vi "IncrementOldHandleMutation.vi"(4 "SerializableData_v2.ctl":path, 6 "Mutate_v1_to_v2.vi":path, 8 "error in (no error)":errorcluster, 10 "Application":refnum<vi>, 11 "LVClassLibrary Ref":refnum<vi>) -> (0 "error out":errorcluster, 2 "Application":refnum<vi>, 3 "LVClassLibrary Ref":refnum<vi>)   [LabVIEW 2019, in "BlueSerializationScripts.lvlib"]
uses:
  BlueSerializationScripts.lvlib
  <userlib>/_OpenG.lib/file/file.llb/File Exists - Scalar__ogtk.vi
  BlueSerialProviderGlobal.vi
  BlueUtilityScripts/BlueUtilityScripts.lvlib
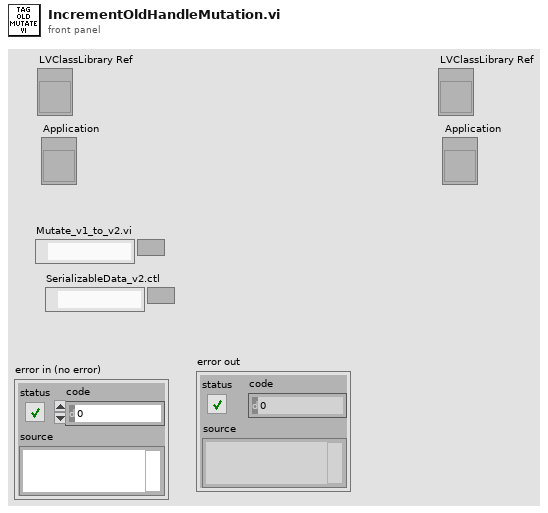
[diagram p1: front panel]
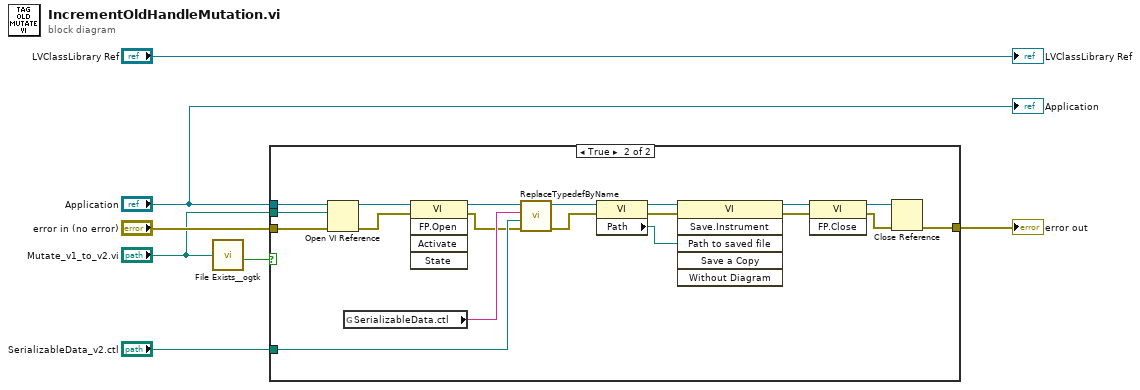
[diagram p0: block diagram]
diagram:
  n1 = call-poly <userlib>:"File Exists__ogtk.vi"("file path"="Mutate_v1_to_v2.vi") -> ("exists"=w1:bool)  [unwired: 6 in, 1 out]
  n2 = case shown="True" w1 {
    tunnel: [w8 w23] -> w7
    tunnel: "Application" -> [_ w22]
    tunnel: "error in (no error)" -> [w8 w21]
    tunnel: "SerializableData_v2.ctl" -> [_ w12]
    tunnel: "Mutate_v1_to_v2.vi" -> [_ w15]
    frame False {
    }
    frame True {
      n3 = Open VI Reference(application reference (local)=w22, vi path=w15, error in (no error)=w21) -> (vi reference=w20:refnum<vi>, error out=w19:errorcluster)  [unwired: 3 in]
      n4 = global read "BlueSerialProviderGlobal.vi" "SerializableData.ctl"() -> (w13:string)
      n5 = invoke class="VI" method="FP.Open"(reference=w20, error in=w19) -> (reference out=w14:refnum<vi>, error out=w10:errorcluster)  [unwired: 3 in, 3 out]
      n6 = call "ReplaceTypedefByName.vi"("error in (no error)"=w10, "Typedef Path"=w12, "Typedef path name"=w13, "VI Refnum"=w14) -> ("error out"=w9:errorcluster, "VI Refnum"=w11:refnum<vi>)  [unwired: 6 in]
      n7 = property class="VI"(reference=w11, error in=w9) -> (reference out=w18:refnum<vi>, error out=w16:errorcluster, "Path"=w17:path)
      n8 = invoke class="VI" method="Save.Instrument"(reference=w18, error in=w16, "Path to saved file"=w17) -> (reference out=w27:refnum<vi>, error out=w26:errorcluster)  [unwired: 3 in, 4 out]
      n9 = invoke class="VI" method="FP.Close"(reference=w27, error in=w26) -> (reference out=w25:refnum<vi>, error out=w24:errorcluster)  [unwired: 1 in, 1 out]
      n10 = Close Reference(reference=w25, error in (no error)=w24) -> (error out=w23:errorcluster)
    }
  }
  "error out" <- w7
  "LVClassLibrary Ref" <- "LVClassLibrary Ref"
  "Application" <- "Application"
